vi "Fill Maps.vi"(10 "Module names":string[](array[string]), 11 "DQMH Modules":refnum<vi>[](array[refnum])) -> (2 "map ref out":map{string, refnum<vi>}(c390), 3 "Tree Map out":T1)   [LabVIEW 2019, in "Panther Dashboard.lvlib"]
uses:
  Panther Dashboard.lvlib
  <vilib>/National Instruments/Tree Map/Tree Map Data.ctl
  Event types--enum.ctl
  <vilib>/National Instruments/Tree Map/Tree Map.lvlib
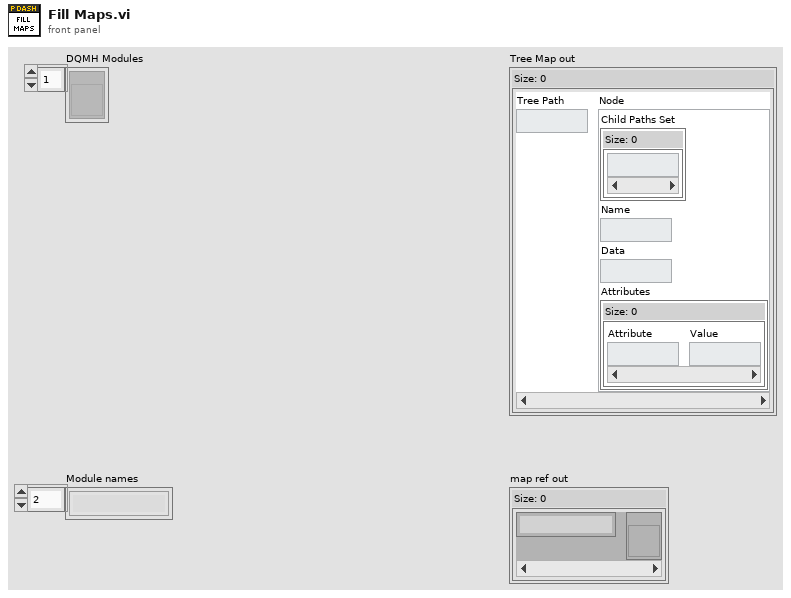
[diagram p1: front panel]
types:
  T1 = typedef "Tree Map.lvlib/Tree Map Data.ctl" = map{string, cluster{"Child Paths Set":set{string}, "Name":string, "Data":string, "Attributes":map{string, string}}}
  T2 = typedef "Panther Dashboard.lvlib/Event types--enum.ctl" = enum16{"Request", "Request and Wait for Reply", "Broadcast"}
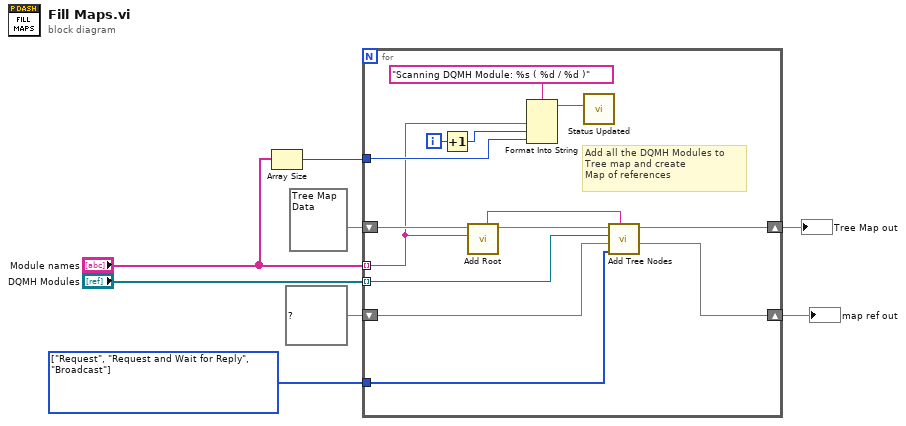
[diagram p0: block diagram]
diagram:
  w4 = T2[] [enum."Request", enum."Request and Wait for Reply", enum."Broadcast"] items=["Request", "Request and Wait for Reply", "Broadcast"] ("Event Types")
  n1 = Array Size(array="Module names") -> (size(s)=w2:i32)
  n2 = for {
    shift-right: [w20] -> w6
    shift-left: T1 {} ("Tree Map out") -> [w11]
    shift-right: [w22] -> w8
    shift-left: map{string, refnum<vi>} {} ("References Map") -> [w21]
    tunnel: "DQMH Modules" -> [w10] mode=indexing
    tunnel: w4 -> [w19]
    tunnel: "Module names" -> [w9] mode=indexing
    tunnel: w2 -> [w17]
    i -> [w18]
    # "Add all the DQMH Modules to\nTree map and create \nMap of references"
    n3 = Increment(x=w18) -> (x+1=w14:i32)
    n4 = call <vilib>:"Add Root.vi"("New Root Name"=w9, "Tree Map In"=w11) -> ("Tree Map Out"=w13:T1, "Root Path"=w12:string)  [unwired: 8 in]
    n5 = Format Into String(format string="Scanning DQMH Module: %s ( %d / %d )", w9, w14, w17) -> (resulting string=w15:string)  [unwired: 2 in, 1 out]
    n6 = call "Status Updated.vi"("Status"=w15) -> ()  [unwired: 10 in, 1 out]
    n7 = call "Add Tree Nodes.vi"("Root path"=w12, "Event Types"=w19, "map ref in"=w21, "DQMH Lib In"=w10, "Tree Map in"=w13) -> ("map ref out"=w22:map{string, refnum<vi>}, "Tree Map out"=w20:T1)  [unwired: 5 in]
  }
  "map ref out" <- w8
  "Tree Map out" <- w6
